vi "Remove AI.vi"(8 "error in (no error)":errorcluster, 10 "Iteration":i32, 11 "Item Ref in":T1 format="%.0x") -> (0 "error out":errorcluster, 3 "Item Ref out":T1 format="%.0x")   [LabVIEW 2020, in "NI PXIe-4340 System Explorer.lvlib"]
doc: "Remove the specified AO channel"
uses:
  NI PXIe-4340 System Explorer.lvlib
  <vilib>/NI VeriStand/Custom Device API/Custom Device Item Ref.ctl
  Shared/Constants.vi
  <vilib>/NI VeriStand/Custom Device API/Get Item Property (Variant).vi
  <vilib>/NI VeriStand/Custom Device API/Custom Device API.lvlib
  Shared/NI PXIe-4340 Shared.lvlib
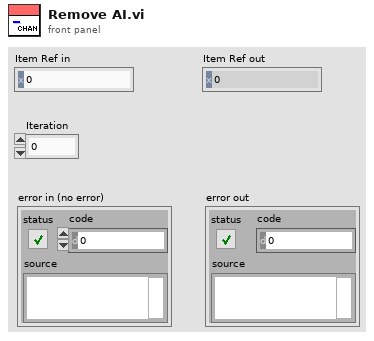
[diagram p1: front panel]
types:
  T1 = typedef "Custom Device API.lvlib/Custom Device Item Ref.ctl" = u64
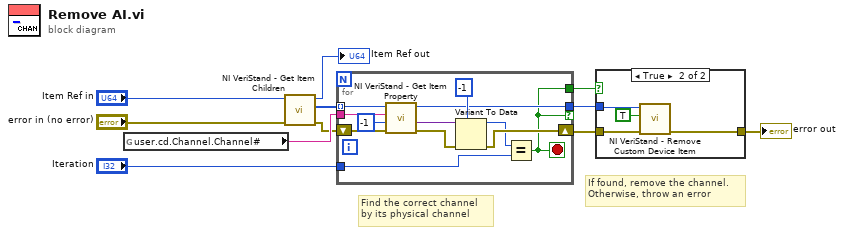
[diagram p0: block diagram]
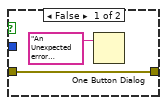
[diagram p2: hidden frame]
diagram:
  # "If found, remove the channel.\nOtherwise, throw an error"
  # "Find the correct channel \nby its physical channel"
  n1 = global read "Constants.vi" "user.cd.Channel.Channel#"() -> (w4:string)
  n2 = call <vilib>:"NI VeriStand - Get Item Children.vi"("error in (no error)"="error in (no error)", "Item Ref in"="Item Ref in") -> ("error out"=w3:errorcluster, "Child Refs"=w2:T1[], "Item Ref out"=→"Item Ref out":T1)  [unwired: 6 in, 1 out]
  n3 = for {
    tunnel: w2 -> [w23] mode=indexing
    shift-right: [w17] -> w9
    shift-left: w3 -> [w22]
    tunnel: w4 -> [w21]
    tunnel: "Iteration" -> [w14]
    tunnel: [w13] -> w7 if=w12
    tunnel: [w12] -> w6
    stop <- w12 stop-if-true
    n4 = call-poly <vilib>:"NI VeriStand - Get Item Property.vi"("error in (no error)"=w22, "Default Value"=-1, "Property Name"=w21, "Item Ref in"=w23) -> ("error out"=w19:errorcluster, "Value"=w18:variant, "Item Ref out"=w13:T1)  [unwired: 4 in, 1 out]
    n5 = Variant To Data(error in=w19, type=-1, Variant=w18) -> (data=w15:i32, error out=w17:errorcluster)
    n6 = Equal?(x=w15, y=w14) -> (x = y?=w12:bool)
  }
  n7 = case shown="True" w6 {
    tunnel: w7 -> [_ w29]
    tunnel: w9 -> [w24 w28]
    tunnel: [w24 w27] -> w10
    frame False {
      n8 = One Button Dialog(message="An Unexpected error occurred. Contact the creator of this device.") -> ()  [unwired: 1 in, 1 out]
    }
    frame True {
      n9 = call <vilib>:"NI VeriStand - Remove Custom Device Item.vi"("error in (no error)"=w28, "Force Delete (F)"=TRUE, "Item Ref in"=w29) -> ("error out"=w27:errorcluster)  [unwired: 7 in, 1 out]
    }
  }
  "error out" <- w10
